vi "IMAQ Pad Image.vi"(6 "Padding Type":T2(ring), 8 "Pixel value (0)":u8, 9 "Pixels":i32, 10 "Image Dest":T1, 11 "Image Src":T1) -> (3 "Image Dest Out":T1)   [LabVIEW 2014]
uses:
  <vilib>/vision/Image Controls.llb/IMAQ Image.ctl
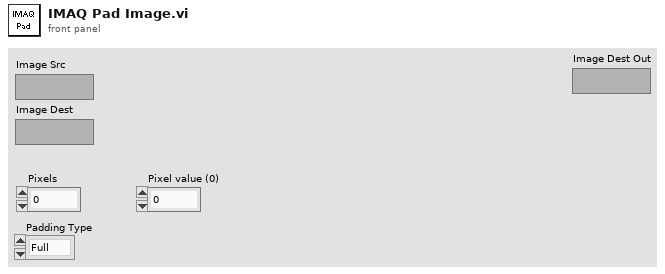
[diagram p1: front panel]
types:
  T1 = typedef "IMAQ Image.ctl" = refnum<image>
  T2 = enum16{"Full", "Left-Top", "Top-Right", "Right-Bottom", "Bottom-Left", "Left", "Top", "Right", "Bottom"}
  T3 = enum16{"Full", "Left-Top", "Top-Right", "Right-Bottom", "Bottom-Left", "Left", "Top", "Right", "Bottom"}[]
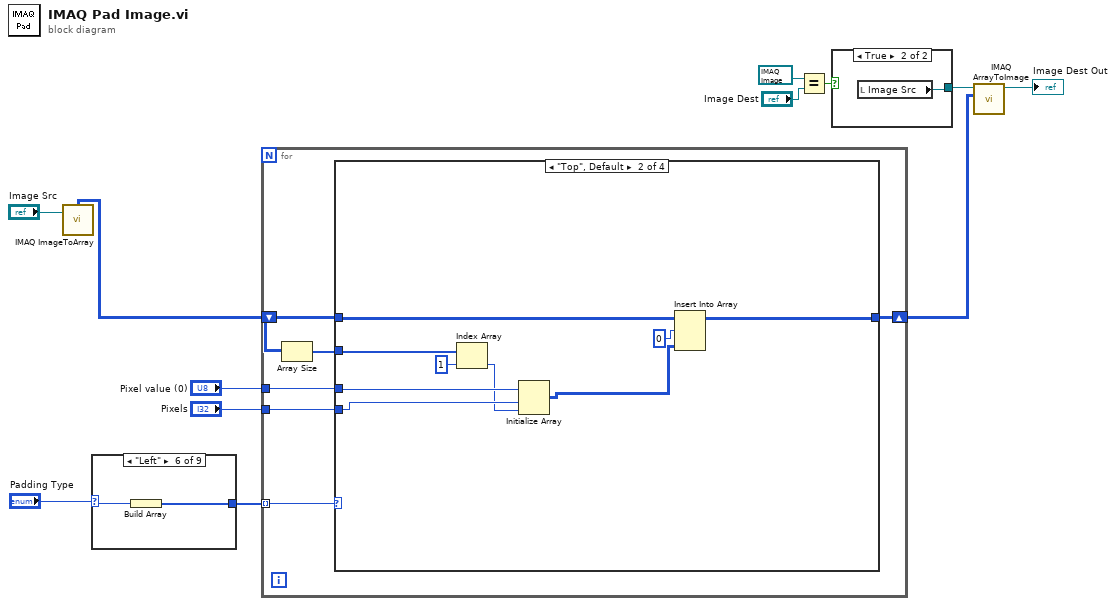
[diagram p0: block diagram]
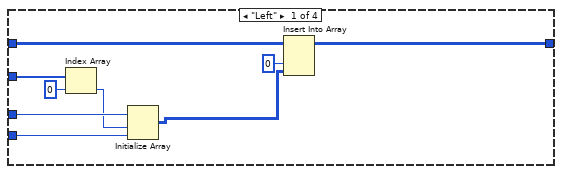
[diagram p2: hidden frame]
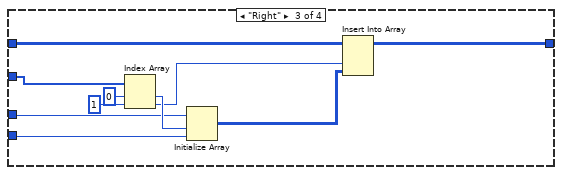
[diagram p3: hidden frame]
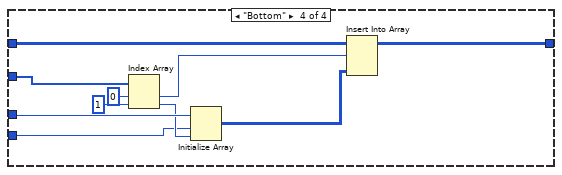
[diagram p4: hidden frame]
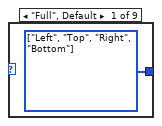
[diagram p5: hidden frame]
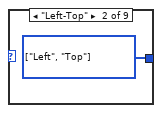
[diagram p6: hidden frame]
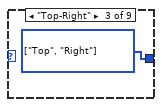
[diagram p7: hidden frame]
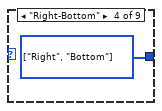
[diagram p8: hidden frame]
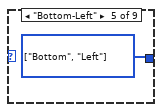
[diagram p9: hidden frame]
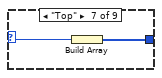
[diagram p10: hidden frame]
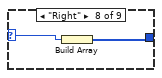
[diagram p11: hidden frame]
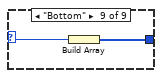
[diagram p12: hidden frame]
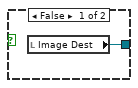
[diagram p13: hidden frame]
diagram:
  n1 = call "IMAQ ImageToArray"("Image"="Image Src") -> ("Image Pixels (U8)"=w4:u8[][])  [unwired: 3 in, 4 out]
  n2 = case shown="\"Left\"" "Padding Type" {
    selector: "Padding Type" -> [_ _ _ _ _ w19 w20 w23 w25]
    tunnel: [w13 w14 w15 w16 w17 w18 w21 w22 w24] -> w5
    frame "Full", Default {
      w13 = T3 [enum."Left", enum."Top", enum."Right", enum."Bottom"] items=["Full", "Left-Top", "Top-Right", "Right-Bottom", "Bottom-Left", "Left", "Top", "Right", "Bottom"]
    }
    frame "Left-Top" {
      w14 = T3 [enum."Left", enum."Top"] items=["Full", "Left-Top", "Top-Right", "Right-Bottom", "Bottom-Left", "Left", "Top", "Right", "Bottom"]
    }
    frame "Top-Right" {
      w15 = T3 [enum."Top", enum."Right"] items=["Full", "Left-Top", "Top-Right", "Right-Bottom", "Bottom-Left", "Left", "Top", "Right", "Bottom"]
    }
    frame "Right-Bottom" {
      w16 = T3 [enum."Right", enum."Bottom"] items=["Full", "Left-Top", "Top-Right", "Right-Bottom", "Bottom-Left", "Left", "Top", "Right", "Bottom"]
    }
    frame "Bottom-Left" {
      w17 = T3 [enum."Bottom", enum."Left"] items=["Full", "Left-Top", "Top-Right", "Right-Bottom", "Bottom-Left", "Left", "Top", "Right", "Bottom"]
    }
    frame "Left" {
      n3 = Build Array(w19) -> (w18:T3)
    }
    frame "Top" {
      n4 = Build Array(w20) -> (w21:T3)
    }
    frame "Right" {
      n5 = Build Array(w23) -> (w22:T3)
    }
    frame "Bottom" {
      n6 = Build Array(w25) -> (w24:T3)
    }
  }
  n7 = for {
    tunnel: w5 -> [w31] mode=indexing
    shift-right: [w26] -> w1
    shift-left: w4 -> [w29]
    tunnel: "Pixel value (0)" -> [w28]
    tunnel: "Pixels" -> [w27]
    n8 = Array Size(array=w29) -> (size(s)=w30:i32[])
    n9 = case shown="\"Top\", Default" w31 {
      tunnel: w30 -> [w40 w46 w55 w65]
      tunnel: w29 -> [w35 w47 w56 w66]
      tunnel: w28 -> [w38 w45 w54 w64]
      tunnel: w27 -> [w33 w44 w53 w62]
      tunnel: [w32 w41 w50 w60] -> w26
      frame "Left" {
        n10 = Index Array(array=w40, index=0) -> (element=w37:i32)
        n11 = Initialize Array(w38, w37, w33) -> (w36:u8[][])
        n12 = Insert Into Array(array=w35, index (col)=0 ("disabled index (col)"), new element=w36) -> (w32:u8[][])  [unwired: 1 in]
      }
      frame "Top", Default {
        n13 = Index Array(array=w46, index=1) -> (element=w43:i32)
        n14 = Initialize Array(w45, w44, w43) -> (w49:u8[][])
        n15 = Insert Into Array(array=w47, index (row)=0 ("disabled index (col)"), new element=w49) -> (w41:u8[][])  [unwired: 1 in]
      }
      frame "Right" {
        n16 = Index Array(array=w55, index #1=0 ("index"), index #2=1 ("index")) -> (element #1=w58:i32, element #2=w51:i32)
        n17 = Initialize Array(w54, w58, w53) -> (w59:u8[][])
        n18 = Insert Into Array(array=w56, index (col)=w51, new element=w59) -> (w50:u8[][])  [unwired: 1 in]
      }
      frame "Bottom" {
        n19 = Index Array(array=w65, index #1=0 ("index"), index #2=1 ("index")) -> (element #1=w61:i32, element #2=w63:i32)
        n20 = Initialize Array(w64, w62, w63) -> (w69:u8[][])
        n21 = Insert Into Array(array=w66, index (row)=w61, new element=w69) -> (w60:u8[][])  [unwired: 1 in]
      }
    }
  }
  n22 = Equal?(x=T1 refnum ("Image Dest"), y="Image Dest") -> (x = y?=w10:bool)
  n23 = case shown="True" w10 {
    tunnel: [w70 w71] -> w9
    frame False {
      n24 = local read "Image Dest"() -> (w70:T1)
    }
    frame True {
      n25 = local read "Image Src"() -> (w71:T1)
    }
  }
  n26 = call "IMAQ ArrayToImage"("Image Pixels (U8)"=w1, "Image"=w9) -> ("Image Out"=→"Image Dest Out":T1)  [unwired: 8 in, 1 out]
